vi "TWO_IMU_logger_2021.vi"(5 "PARAMETERS":dbl[](array[numeric])=[1.0, 2.0, 3.0], 6 "Folder":path, 7 "LOG":bool, 10 "DATA":dbl[][](array[numeric])) -> (8 "FileName":string)   [LabVIEW 2021]
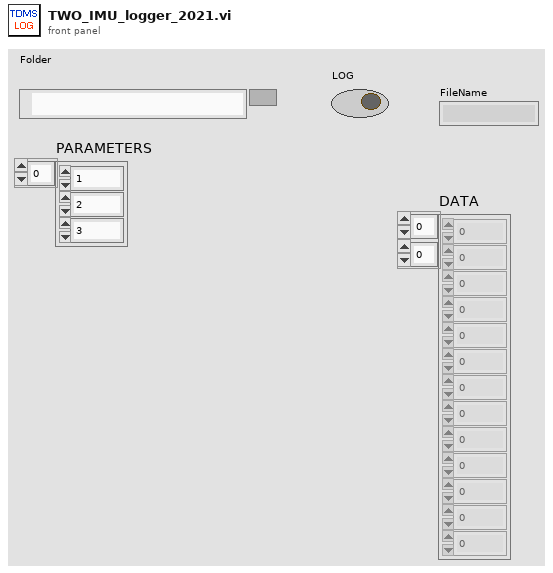
[diagram p1: front panel]
types:
  T1 = enum16{"open", "open or create", "create or replace", "create", "open (read-only)"}
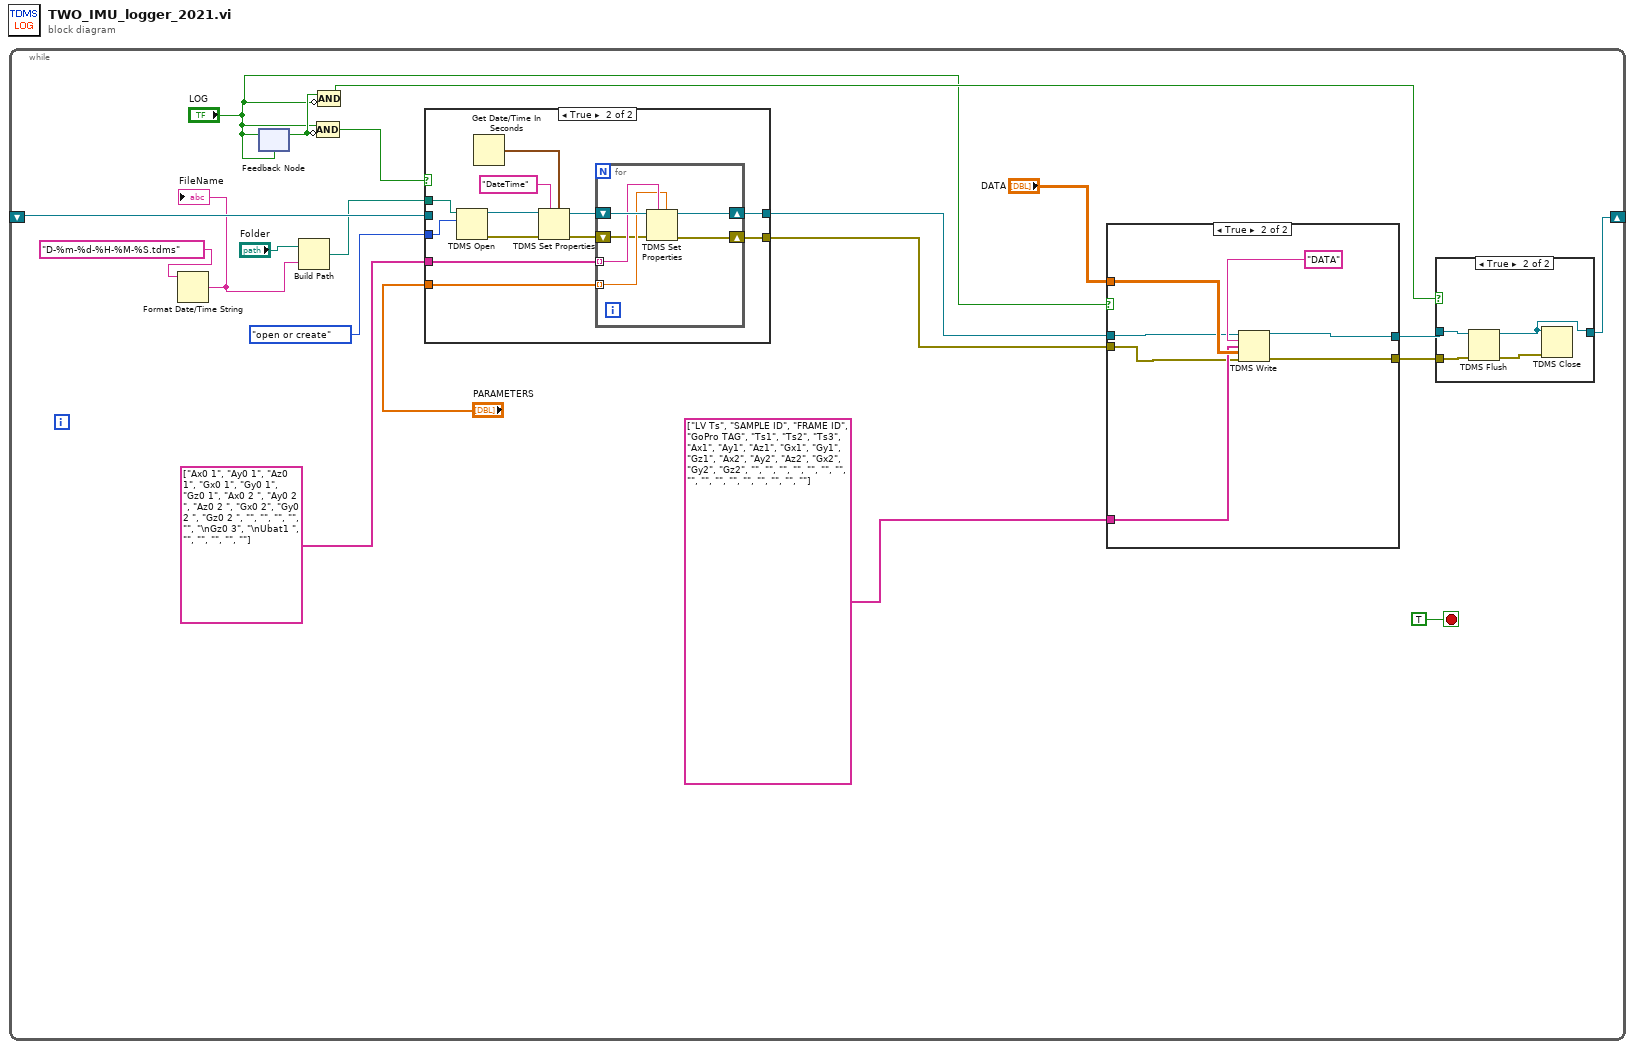
[diagram p0: block diagram]
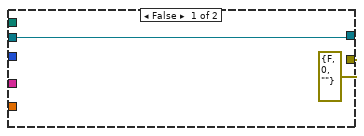
[diagram p3: hidden frame]
diagram:
  n1 = while {
    shift-right: [w6] -> _
    shift-left: _ -> [w20]
    stop <- TRUE stop-if-true
    n2 = Format Date/Time String(time format string (%c)="D-%m-%d-%H-%M-%S.tdms") -> (date/time string=w11:string)  [unwired: 2 in]
    "FileName" <- w11
    n3 = feedback-in #1("LOG") -> ()
    n4 = feedback #1("LOG") -> (w19:bool)
    n5 = Build Path(base path="Folder", name or relative path=w11) -> (appended path=w2:path)
    n6 = Compound Arithmetic op=AND("LOG", invert w19) -> (w3:bool)
    n7 = Compound Arithmetic op=AND(w19, invert "LOG") -> (w18:bool)
    n8 = case shown="True" w3 {
      tunnel: [w31 w38] -> w16
      tunnel: w20 -> [w31 _]
      tunnel: w2 -> [_ w32]
      tunnel: T1."open or create" ("operation (0:open)") -> [_ w43]
      tunnel: string[] ["Ax0 1", "Ay0 1", "Az0 1", "Gx0 1", "Gy0 1", "Gz0 1", "Ax0 2 ", "Ay0 2 ", "Az0 2 ", "Gx0 2", "Gy0 2 ", "Gz0 2 ", "", "", "", "", "", "\nGz0 3", "\nUbat1 ", "", "", "", "", ""] -> [_ w37]
      tunnel: "PARAMETERS" -> [_ w36]
      tunnel: [errorcluster {"status"=FALSE, "code"=0, "source"=""} ("error out") w33] -> w7
      frame False {
      }
      frame True {
        n9 = TDMS Open(10:w43, 11:w32) -> (0:w35:errorcluster, 3:w42:refnum<k34>)  [unwired: 5 in]
        n10 = Get Date/Time In Seconds() -> (seconds since 1Jan1904=w40:timestamp)
        n11 = TDMS Set Properties(5:w40, 7:"DateTime", 8:w35, 11:w42) -> (0:w34:errorcluster, 3:w39:refnum<k34>)  [unwired: 2 in, 2 out]
        n12 = for {
          shift-right: [w48] -> w38
          shift-left: w39 -> [w49]
          tunnel: w37 -> [w47] mode=indexing
          tunnel: w36 -> [w46] mode=indexing
          shift-right: [w44] -> w33
          shift-left: w34 -> [w45]
          n13 = TDMS Set Properties(5:w46, 7:w47, 8:w45, 11:w49) -> (0:w44:errorcluster, 3:w48:refnum<k34>)  [unwired: 2 in, 2 out]
        }
      }
    }
    n14 = case shown="True" "LOG" {
      tunnel: w16 -> [w22 w24]
      tunnel: [w22 w25] -> w5
      tunnel: string[] ["LV Ts", "SAMPLE ID", "FRAME ID", "GoPro TAG", "Ts1", "Ts2", "Ts3", "Ax1", "Ay1", "Az1", "Gx1", "Gy1", "Gz1", "Ax2", "Ay2", "Az2", "Gx2", "Gy2", "Gz2", "", "", "", "", "", "", "", "", "", "", "", "", "", "", "", ""] ("channel name(s) in (Untitled)") -> [_ w27]
      tunnel: "DATA" -> [_ w28]
      tunnel: w7 -> [w21 w23]
      tunnel: [w21 w26] -> w4
      frame False {
      }
      frame True {
        n15 = TDMS Write(0:w24, 5:"DATA" ("group name in (Untitled)"), 7:w27, 9:w28, 11:w23) -> (4:w25:refnum<k34>, 15:w26:errorcluster)  [unwired: 1 in, 2 out]
      }
    }
    n16 = case shown="True" w18 {
      tunnel: w5 -> [w50 w54]
      tunnel: [w50 w51] -> w6
      tunnel: w4 -> [_ w53]
      frame False {
      }
      frame True {
        n17 = TDMS Flush(4:w53, 7:w54) -> (0:w52:errorcluster, 3:w51:refnum<k34>)
        n18 = TDMS Close(8:w52, 11:w51) -> ()  [unwired: 2 out]
      }
    }
  }
